vi "age sub vi.vi"(4 "birth\nday":dbl, 6 "current\nday":dbl, 7 "current\nyear":dbl, 9 "birth\nmonth":dbl, 10 "Current\nmonth":dbl, 11 "birth\nyear":dbl) -> (3 "age":dbl)   [LabVIEW 2018]
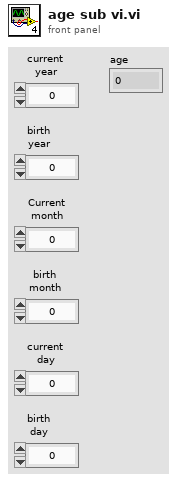
[diagram p1: front panel]
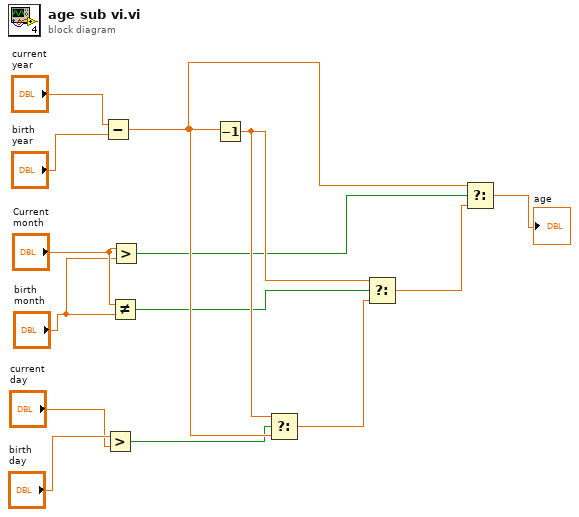
[diagram p0: block diagram]
diagram:
  n1 = Subtract(x="current\nyear", y="birth\nyear") -> (x-y=w10:dbl)
  n2 = Greater?(x="birth\nday", y="current\nday") -> (0:w7:bool)
  n3 = Not Equal?(x="Current\nmonth", y="birth\nmonth") -> (x != y?=w9:bool)
  n4 = Greater?(x="Current\nmonth", y="birth\nmonth") -> (0:w8:bool)
  n5 = Decrement(x=w10) -> (x-1=w11:dbl)
  n6 = Select(t=w11, s=w7, f=w10) -> (s? t:f=w12:dbl)
  n7 = Select(t=w11, s=w9, f=w12) -> (s? t:f=w13:dbl)
  n8 = Select(t=w10, s=w8, f=w13) -> (s? t:f=→"age":dbl)
